vi "OOP_DOWN.vi"(8 "error in (no error)":errorcluster, 10 "Sett data":T2={"Filter"=4, "Gain"=4.0, "Bit rate"=4.0, "ISO/IEC w "=enum."14443 Type A", "BI"={"R"=0.0, "C"=0.0, "L"=0.0}, "BM"={"R"=0.0, "C"=0.0, "L"=0.0}, "M"={"Метка"=4, "Считыветель"=4}, "Type noise"=enum."Гауссовский шум", "Link"=enum."UPLINK", "Noise attenuator"=0.0, "Signal gain"=1.0, "Distance"=0.0} {"Distance" scale=0.0..10.0; "Signal gain" min=1.0 max=100.0 step=1.0 scale=1.0..30.0; "Noise attenuator" scale=0.01..1.01; "M"."Считыветель" min=4 max=128 step=4; "M"."Метка" min=4 max=128 step=4; "Bit rate" min=4.0 max=128.0 step=4.0; "Gain" min=4.0 max=128.0 step=4.0; "Filter" min=4 max=128 step=4}, 11 "RFID system.lvclass":refnum<class "RFID system.lvclass">) -> (0 "error out":errorcluster, 2 "Error on  byte":dbl, 3 "Visual":T1={"Notes"=[], "Frame"=[1]}, 5 "Power out":waveform(dbl))   [LabVIEW 2019]
uses:
  Class/RFID system.lvclass
  TypeDef/Sett data.ctl
  TypeDef/ISO.ctl
  TypeDef/Noise.ctl
  TypeDef/Link.ctl
  UI/Visual/data.ctl
  TypeDef/Store.ctl
  UI/Visual/Visual.xctl
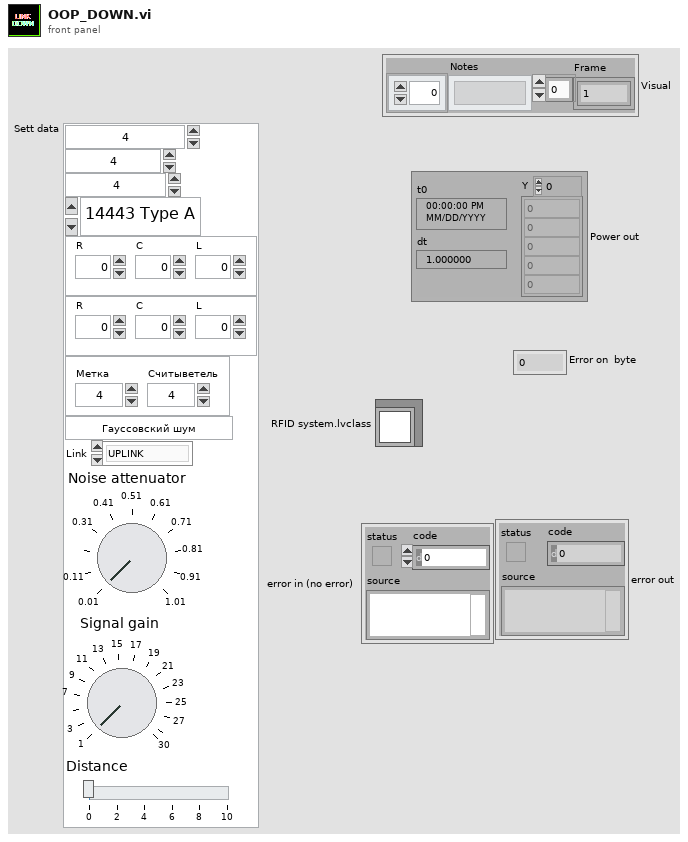
[diagram p1: front panel]
types:
  T1 = typedef "Visual.xctl/data.ctl" = cluster{"Notes":string[], "Frame":u8[]}
  T2 = typedef "Sett data.ctl" = cluster{"Filter":i32, "Gain":dbl, "Bit rate":dbl, "ISO/IEC w ":T3, "BI":cluster{"R":dbl, "C":dbl, "L":dbl}, "BM":cluster{"R":dbl, "C":dbl, "L":dbl}, "M":cluster{"Метка":i64, "Считыветель":i64}, "Type noise":T4, "Link":T5, "Noise attenuator":dbl, "Signal gain":dbl, "Distance":dbl}
  T3 = typedef "ISO.ctl" = enum16{"14443 Type A", "14443 Type B", "Felica", "15693"}
  T4 = typedef "Noise.ctl" = enum16{"Гауссовский шум", "Белый шум"}
  T5 = typedef "Link.ctl" = enum16{"UPLINK", "DOWNLINK"}
  T6 = typedef "Store.ctl" = enum16{"envelope", "noise", "demSubCar", "CH_frame", "Decode", "demodulate", "in", "out", "sum", "subCarrier", "frame", "command", "encode", "modulate", "encode_UP", "modulate_up", "demod_up", "envelop_up", "sum_up", "out_up", "in_up"}
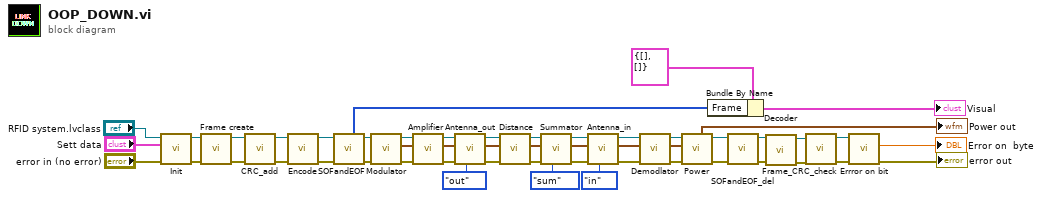
[diagram p0: block diagram]
diagram:
  n1 = call "Init.vi"("error in (no error)"="error in (no error)", "Sett data"="Sett data", "RFID system in"="RFID system.lvclass") -> ("error out"=w51:errorcluster, "RFID system out"=w50:refnum<class "RFID system.lvclass">)  [unwired: 7 in]
  n2 = call-dynamic "Frame create.vi"("error in (no error)"=w51, "RFID system in"=w50) -> ("error out"=w49:errorcluster, "RFID system out"=w48:refnum<class "RFID system.lvclass">)  [unwired: 8 in]
  n3 = call-dynamic "CRC_add.vi"("error in (no error)"=w49, "RFID system in"=w48) -> ("error out"=w9:errorcluster, "RFID system out"=w10:refnum<class "RFID system.lvclass">)  [unwired: 8 in]
  n4 = call-dynamic "Encode.vi"("error in (no error)"=w9, "RFID system in"=w10) -> ("error out"=w11:errorcluster, "RFID system out"=w12:refnum<class "RFID system.lvclass">)  [unwired: 8 in]
  n5 = call-dynamic "SOFandEOF.vi"("error in (no error)"=w11, "RFID system in"=w12) -> ("error out"=w7:errorcluster, "RFID system out"=w8:refnum<class "RFID system.lvclass">, "frame"=w16:u8[])  [unwired: 7 in]
  n6 = call-dynamic "Modulator.vi"("error in (no error)"=w7, "RFID system in"=w8) -> ("error out"=w46:errorcluster, "Waveform out"=w43:waveform(dbl), "RFID system out"=w47:refnum<class "RFID system.lvclass">)  [unwired: 7 in]
  n7 = call "Amplifier.vi"("error in (no error)"=w46, "Waveform in"=w43, "RFID system in"=w47) -> ("error out"=w44:errorcluster, "Waveform out"=w42:waveform(dbl), "RFID system out"=w45:refnum<class "RFID system.lvclass">)  [unwired: 6 in]
  n8 = call "Antenna_out.vi"("Store"=Store."out", "error in (no error)"=w44, "Waveform in"=w42, "RFID system in"=w45) -> ("error out"=w24:errorcluster, "Waveform out"=w26:waveform(dbl), "RFID system out"=w25:refnum<class "RFID system.lvclass">)  [unwired: 5 in]
  n9 = call "Distance.vi"("error in (no error)"=w24, "Waveform in"=w26, "RFID system in"=w25) -> ("error out"=w23:errorcluster, "Waveform out"=w22:waveform(dbl), "RFID system out"=w21:refnum<class "RFID system.lvclass">)  [unwired: 6 in]
  n10 = call "Summator.vi"("Store"=Store."sum", "error in (no error)"=w23, "Waveform in"=w22, "RFID system in"=w21) -> ("error out"=w18:errorcluster, "Waveform out"=w19:waveform(dbl), "RFID system out"=w20:refnum<class "RFID system.lvclass">)  [unwired: 5 in]
  n11 = call "Antenna_in.vi"("Store"=Store."in", "error in (no error)"=w18, "Waveform in"=w19, "RFID system in"=w20) -> ("error out"=w35:errorcluster, "Waveform out"=w34:waveform(dbl), "RFID system out"=w36:refnum<class "RFID system.lvclass">)  [unwired: 5 in]
  n12 = call-dynamic "Demodlator.vi"("error in (no error)"=w35, "Waveform in"=w34, "RFID system in"=w36) -> ("error out"=w31:errorcluster, "Waveform out"=w14:waveform(dbl), "RFID system out"=w30:refnum<class "RFID system.lvclass">)  [unwired: 6 in]
  n13 = call "Power.vi"("error in (no error)"=w31, "Waveform in"=w14, "RFID system in"=w30) -> ("error out"=w5:errorcluster, "RFID system out"=w6:refnum<class "RFID system.lvclass">, "Waveform out"=→"Power out":waveform(dbl))  [unwired: 6 in]
  n14 = Bundle By Name(cluster=T1 {"Notes"=[], "Frame"=[]} ("Store"), "Frame"=w16) -> (→"Visual":T1)
  n15 = call-dynamic "SOFandEOF_del.vi"("error in (no error)"=w5, "RFID system in"=w6) -> ("error out"=w4:errorcluster, "RFID system out"=w3:refnum<class "RFID system.lvclass">)  [unwired: 8 in]
  n16 = call-dynamic "Decoder.vi"("error in (no error)"=w4, "RFID system in"=w3) -> ("error out"=w1:errorcluster, "RFID system out"=w2:refnum<class "RFID system.lvclass">)  [unwired: 8 in]
  n17 = call-dynamic "Frame_CRC_check.vi"("error in (no error)"=w1, "RFID system in"=w2) -> ("error out"=w33:errorcluster, "RFID system out"=w32:refnum<class "RFID system.lvclass">)  [unwired: 8 in]
  n18 = call-dynamic "Errror on bit.vi"("error in (no error)"=w33, "RFID system in"=w32) -> ("error out"=→"error out":errorcluster, "Error on  byte"=→"Error on  byte":dbl)  [unwired: 7 in, 1 out]
